vi "RSZVB Get Signal Power Mode.vi"(8 "error in (no error)":errorcluster {"code" format="%.0x"}, 9 "Signal (RF)":i32(ring) items=["RF"=0, "IF"=2, "LO 1"=3, "LO 2"=4, "Aux LO"=5], 10 "Channel (1)":i32=1, 11 "VISA resource name":refnum<visa-resource-name>) -> (0 "error out":errorcluster {"code" format="%.0x"}, 2 "Mode":i32, 3 "VISA resource name out":refnum<visa-resource-name>)   [LabVIEW 2011]
doc: "This VI queries if the RF, LO 1, LO 2, Aux LO, or the IF signal ports are set to fixed power or to the channel base power.\n\nRemote-control command(s):\nSOURce<Ch>:FREQuency<Pt>:CONVersion:MIXer:PMODe? RF | LO | LO1 | LO2 | AUXLo | IF"
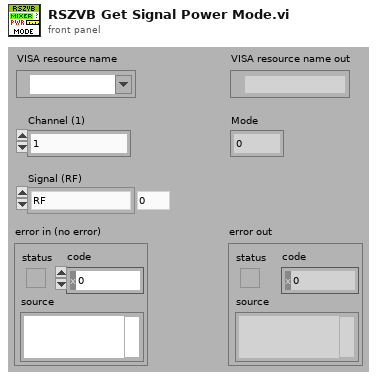
[diagram p1: front panel]
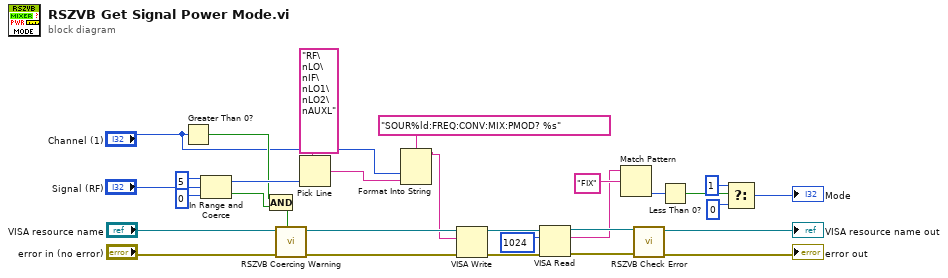
[diagram p0: block diagram]
diagram:
  n1 = Greater Than 0?(x="Channel (1)") -> (x > 0?=w20:bool)
  n2 = In Range and Coerce(upper limit=5, x="Signal (RF)", lower limit=0) -> (coerced(x)=w24:i32, In Range?=w19:bool)
  n3 = Compound Arithmetic op=AND(w20, w19) -> (w28:bool)
  n4 = call "RSZVB Coercing Warning.vi"("In Range?"=w28, "error in (no error)"="error in (no error)", "VISA session"="VISA resource name") -> ("error out"=w29:errorcluster, "dup VISA session"=w30:refnum<visa-resource-name>)  [unwired: 7 in]
  n5 = Pick Line(multi-line string="RF\nLO\nIF\nLO1\nLO2\nAUXL", line index=w24) -> (output string=w21:string)  [unwired: 1 in]
  n6 = Format Into String(format string="SOUR%ld:FREQ:CONV:MIX:PMOD? %s", "Channel (1)", w21) -> (resulting string=w26:string)  [unwired: 2 in, 1 out]
  n7 = VISA Write(VISA resource name=w30, write buffer=w26, error in (no error)=w29) -> (VISA resource name out=w11:refnum<visa-resource-name>, error out=w10:errorcluster)  [unwired: 1 out]
  n8 = VISA Read(VISA resource name=w11, byte count=u32 1024 ("byte count (0)"), error in (no error)=w10) -> (VISA resource name out=w9:refnum<visa-resource-name>, read buffer=w1:string, error out=w8:errorcluster)  [unwired: 1 out]
  n9 = Match Pattern(string=w1, regular expression="FIX") -> (offset past match=w12:i32)  [unwired: 1 in, 3 out]
  n10 = call "RSZVB Check Error.vi"("error in (no error)"=w8, "VISA session"=w9) -> ("error out"=→"error out":errorcluster, "dup VISA session"=→"VISA resource name out":refnum<visa-resource-name>)  [unwired: 8 in]
  n11 = Less Than 0?(x=w12) -> (x < 0?=w6:bool)
  n12 = Select(t=1, s=w6, f=0 ("byte count (0)")) -> (s? t:f=→"Mode":i32)
